vi "fisheye_camera_poly1.vi"(0 "Fisheye Camera configuration":string="{\n    \"type\": \"Poly1FisheyeCamera\",\n   \t\"listen_port\": 8018,\n   \t\"description\": \"\",  \n    \"location\": {\n\t\t  \"x\": 0.0,\n\t\t  \"y\": 0.0,\n\t\t  \"z\": 225.0\n\t},\n    \"stream_dimensions\": {\n\t\t      \"x\": 512,\n\t\t     \"y\": 512\n\t},\n    \"rotation\": {\n\t\t      \"pitch\": 0.0,\n\t\t      \"roll\": 0.0,\n\t\t      \"yaw\": 0.0\n\t},\n    \"viewport\": {\n\t\t      \"enable_viewport\": false,\n\t\t      \"fullscreen\": false,\n\t\t      \"monitor_name\": \"\",\n\t\t      \"monitor_number\": 0,\n        \"window_offset\": {\n\t\t\t         \"x\": 32,\n\t\t\t         \"y\": 32\n  \t\t},\n\t\t     \"window_size\": {\n\t\t         \"x\": 0,\n\t\t\t        \"y\": 0\n\t\t      }\n\t},\n\t\"a0\": 350,\n\t\"a2\": -0.001,\n\t\"a3\": 1.2e-06,\n\t\"a4\": -1.5e-09,\n \"ray_tracing\":{\n        \"enable_ray_tracing\": false\n     },\n\t\"channel_depth\": 1,\n\t\"channels\": \"bgra\",\n\t\"dynamic_range\": 50.0,\n\t\"enable_streaming\": true,\n\t\"face_size\": 492,\n\t\"focal_length\": 9.0,\n\t\"fov\": 180.0,\n\t\"fstop\": 1.399999976158142,\n\t\"max_distance\": 50000.0,\n\t\"max_shutter\": 0.00139999995008111,\n\t\"min_shutter\": 0.0005000000237487257,\n\t\"sensor_size\": 9.069999694824219,\n\t\"wait_for_fresh_frame\": true\n}", 3 "error In":errorcluster={"status"=FALSE, "code"=0, "source"="\"complete\","}) -> (4 "Camera configuration":string="{\n    \"type\": \"Poly1FisheyeCamera\",\n   \t\"listen_port\": 8018,\n   \t\"description\": \"\",  \n    \"location\": {\n\t\t  \"x\": 0.0,\n\t\t  \"y\": 0.0,\n\t\t  \"z\": 225.0\n\t},\n    \"stream_dimensions\": {\n\t\t      \"x\": 512,\n\t\t     \"y\": 512\n\t},\n    \"rotation\": {\n\t\t      \"pitch\": 0.0,\n\t\t      \"roll\": 0.0,\n\t\t      \"yaw\": 0.0\n\t},\n    \"viewport\": {\n\t\t      \"enable_viewport\": false,\n\t\t      \"fullscreen\": false,\n\t\t      \"monitor_name\": \"\",\n\t\t      \"monitor_number\": 0,\n        \"window_offset\": {\n\t\t\t         \"x\": 0,\n\t\t\t         \"y\": 0\n  \t\t},\n\t\t     \"window_size\": {\n\t\t         \"x\": 0,\n\t\t\t        \"y\": 0\n\t\t      }\n\t},\n\t\"a0\": 349.1260070800781,\n\t\"a2\": -0.0010999999940395355,\n\t\"a3\": 1.1977999747614376e-06,\n\t\"a4\": -1.5119000496000012e-09,\n\t\"channel_depth\": 1,\n\t\"channels\": \"bgra\",\n\t\"dynamic_range\": 50.0,\n\t\"enable_streaming\": true,\n\t\"face_size\": 492,\n\t\"focal_length\": 9.0,\n\t\"fov\": 180.0,\n\t\"fstop\": 1.399999976158142,\n\t\"max_distance\": 50000.0,\n\t\"max_shutter\": 0.00139999995008111,\n\t\"min_shutter\": 0.0005000000237487257,\n\t\"sensor_size\": 9.069999694824219,\n\t\"wait_for_fresh_frame\": true\n}", 5 "Image":picture, 6 "Raw data":u8[](array[numeric]), 8 "error out":errorcluster)   [LabVIEW 2019]
doc: "Configures and reads the data stream for a Fisheye Camera, this camera is a scaramuzza model based."
uses:
  controls/Header.ctl
  tools/simx_common.vi
panel:
  in  "camera_connection":refnum<k5>
  in  "null connection":refnum<k5>
  out "Header":T1 {"game_time" format="%_10g"}
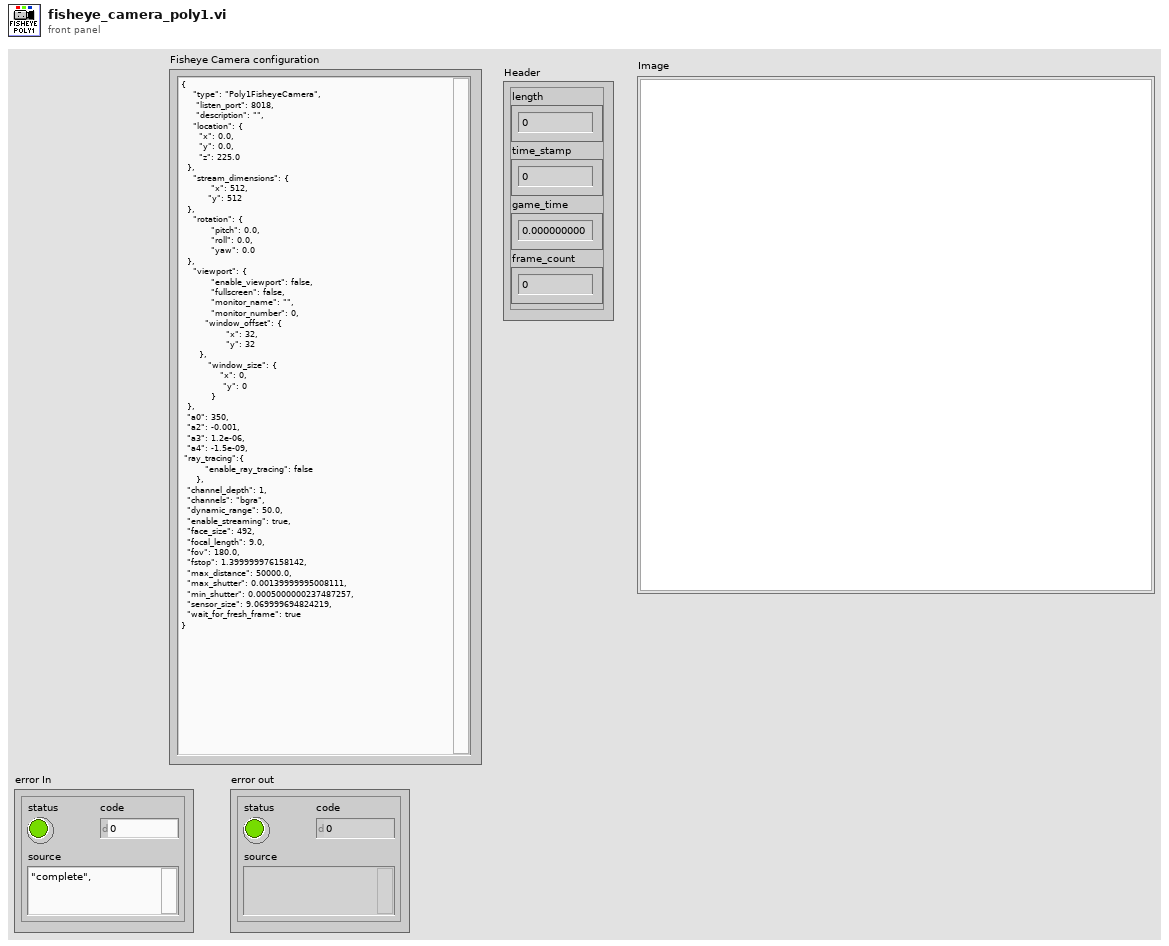
[diagram p1: front panel]
types:
  T1 = typedef "Header.ctl" = cluster{"length":u32, "time_stamp":u32, "game_time":sgl, "frame_count":u32}
  T2 = typedef "simx_connection.ctl" = cluster{"Config":T3, "Connections":T6, "Map":cluster{"lanes":cluster{"x":dbl[], "y":dbl[], "z":dbl[]}, "StartPosition":cluster{"start_points":T7, "StartRotation":dbl[], "StartLocation":dbl[]}, "Draw Map Size":T8, "DrawArea":cluster{"min_Y":dbl, "min_X":dbl, "Scale X":dbl, "Scale Y":dbl}, "Map":picture, "Map Geojson":string}}
  T3 = typedef "config.ctl" = cluster{"Trajectory":T4, "Weather":T5}
  T4 = typedef "trajectory.ctl" = cluster{"Number of frames":i32, "Frame number":i32, "Trajectory":string}
  T5 = typedef "weather.ctl" = cluster{"id":string}
  T6 = typedef "connections.ctl" = cluster{"Simulator Connection":refnum<k5>, "server_ip":string, "Port":i32, "Sensor connections":refnum<k5>[]}
  T7 = typedef "start_points.ctl" = cluster{"locations":dbl[][], "rotations":dbl[][], "type":string[]}
  T8 = typedef "LVBoundsTypeDef.ctl" = cluster{"Width":u32, "Height":u32}
  T9 = typedef "sensor_sample.ctl" = cluster{"Header":T1, "data out":string}
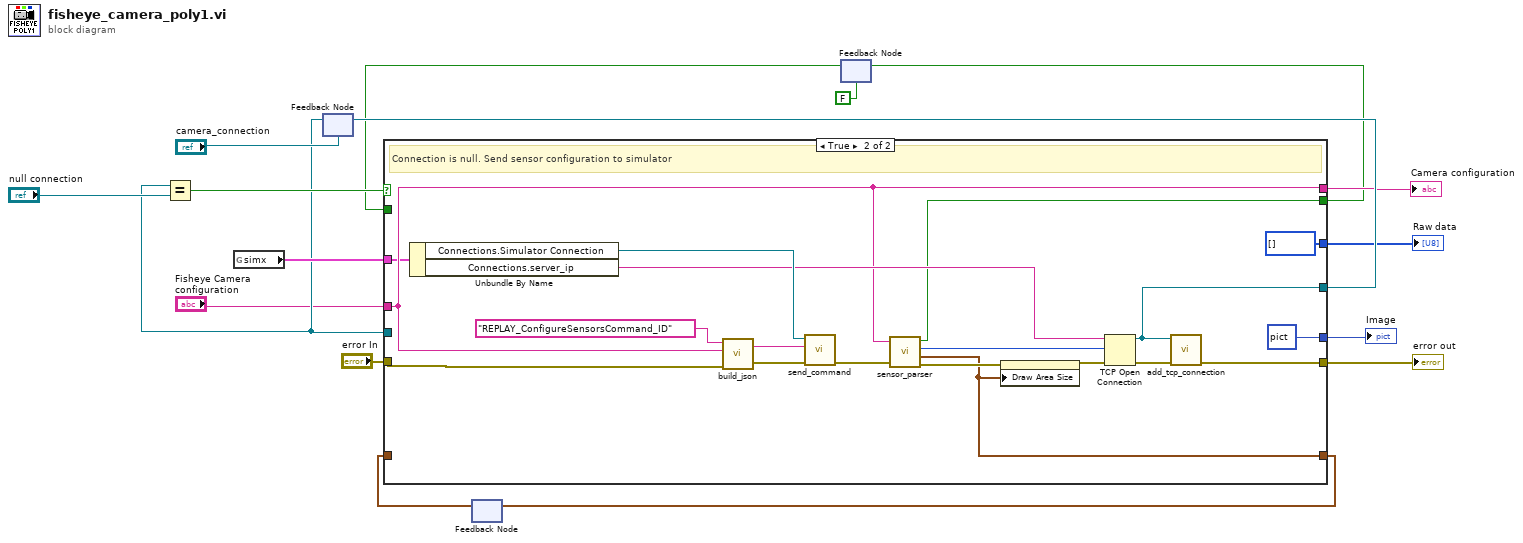
[diagram p0: block diagram]
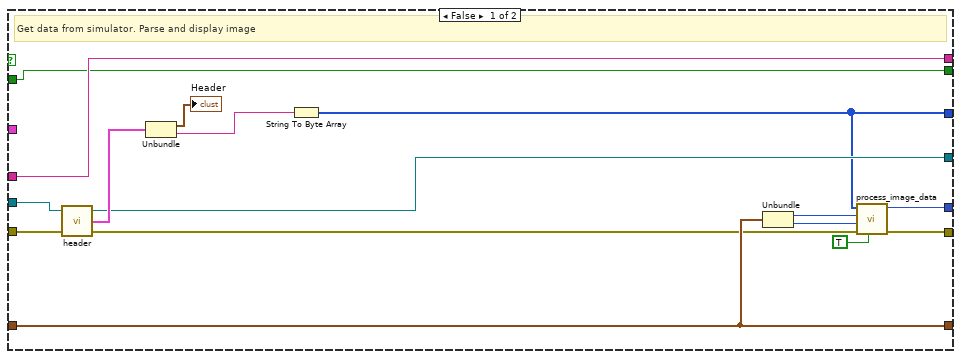
[diagram p2: hidden frame]
diagram:
  n1 = global read "simx_common.vi" "simx"() -> (w3:T2)
  n2 = feedback #1("camera_connection") -> (w2:refnum<k5>)
  n3 = Equal?(x=w2, y="null connection") -> (x = y?=w15:bool)
  n4 = feedback #2() -> (w10:cluster{"x dimension":i32, "y dimension":i32})  [unwired: 1 in]
  n5 = feedback #3(FALSE) -> (w4:bool)
  n6 = case shown="True" w15 {
    tunnel: [w24 w34] -> w13
    tunnel: "Fisheye Camera configuration" -> [w28 w38]
    tunnel: [w25 w36] -> w16
    tunnel: w2 -> [w31 _]
    tunnel: "error In" -> [w30 w44]
    tunnel: w10 -> [w29 _]
    tunnel: [w19 picture data[5B] ("new picture")] -> w7
    tunnel: [w29 w41] -> w11
    tunnel: [w22 u8[] [] ("unsigned byte array")] -> w9
    tunnel: [w28 w38] -> w8
    tunnel: [w27 w40] -> w6
    tunnel: w4 -> [w27 _]
    tunnel: w3 -> [_ w37]
    frame False {
      # "Get data from simulator. Parse and display image"
      n7 = call "header.vi"("error in"=w30, "TCP Network Connection in"=w31) -> ("error out"=w23:errorcluster, "Sensor sample"=w32:T9, "TCP Network Connection out"=w25:refnum<k5>)  [unwired: 1 in]
      n8 = Unbundle(w32) -> ("Header"=→"Header":T1, "data out"=w33:string)
      n9 = String To Byte Array(string=w33) -> (unsigned byte array=w22:u8[])
      n10 = Unbundle(w29) -> ("x dimension"=w21:i32, "y dimension"=w20:i32)
      n11 = call "process_image_data.vi"("RGBA"=TRUE, "error in"=w23, "y"=w20, "x"=w21, "Raw data"=w22) -> ("error out"=w24:errorcluster, "Image"=w19:picture)  [unwired: 3 in]
    }
    frame True {
      # "Connection is null. Send sensor configuration to simulator"
      n12 = Unbundle By Name(w37) -> ("Connections.Simulator Connection"=w47:refnum<k5>, "Connections.server_ip"=w45:string)
      n13 = call "build_json.vi"("error in"=w44, "Message"=w38, "Command_ID"="REPLAY_ConfigureSensorsCommand_ID") -> ("error out"=w50:errorcluster, "JSON Out"=w51:string)  [unwired: 1 in]
      n14 = call "send_command.vi"("error in"=w50, "JSON Command"=w51, "TCP Network Connection in"=w47) -> ("error out"=w43:errorcluster)  [unwired: 1 in, 3 out]
      n15 = call "sensor_parser.vi"("Sensor configuration"=w38, "error in"=w43) -> ("include_annotation"=w40:bool, "Port out"=w39:u16, "Stream dimensions"=w41:cluster{"x dimension":i32, "y dimension":i32}, "error out"=w42:errorcluster)  [unwired: 1 in]
      n16 = property on="Image" class="Pict"(error in=w42, "Draw Area Size"=w41) -> (error out=w46:errorcluster)  [unwired: 1 in, 1 out]
      n17 = TCP Open Connection(address=w45, remote port or service name=w39, error in (no error)=w46) -> (connection ID=w36:refnum<k5>, error out=w35:errorcluster)  [unwired: 2 in]
      n18 = call "add_tcp_connection.vi"("error in"=w35, "Sensor connection"=w36) -> ("error out"=w34:errorcluster)  [unwired: 5 in]
    }
  }
  "error out" <- w13
  "Image" <- w7
  "Raw data" <- w9
  "Camera configuration" <- w8
  n19 = feedback-in #1(w16) -> ()
  n20 = feedback-in #2(w11) -> ()
  n21 = feedback-in #3(w6) -> ()
